vi "Communicate with Simulated Temperature Control.vi"(5 "error in (no error)":errorcluster, 6 "stop":bool, 7 "Setpoint":dbl=20.0 format="%.2f", 8 "connection ID":refnum<k5>) -> (0 "error out":errorcluster, 1 "Temperature":dbl(slide) scale=0.0..100.0, 2 "Stabilized":bool, 3 "connection ID Out":refnum<k5>)   [LabVIEW 2010]
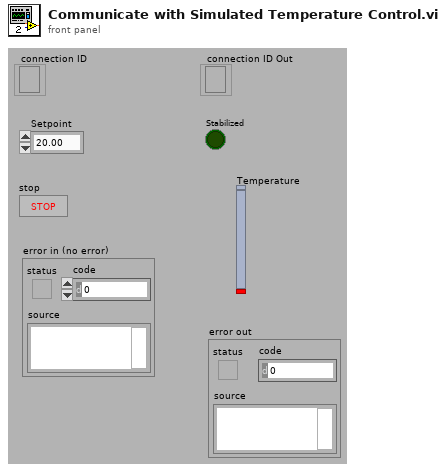
[diagram p1: front panel]
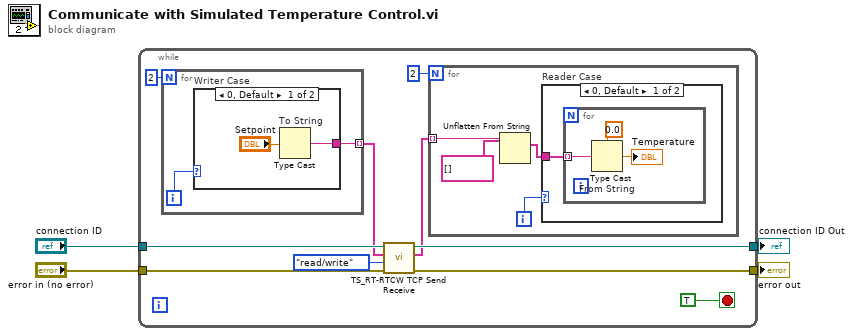
[diagram p0: block diagram]
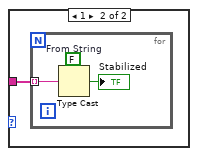
[diagram p2: hidden frame]
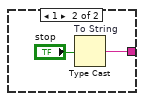
[diagram p3: hidden frame]
diagram:
  n1 = while {
    tunnel: [w13] -> w2
    tunnel: "connection ID" -> [w12]
    tunnel: "error in (no error)" -> [w14]
    tunnel: [w9] -> w4
    stop <- TRUE stop-if-true
    n2 = for {
      N: 2 -> [_]
      tunnel: [w27] -> w10 mode=indexing
      i -> [w28]
      n3 = case "Writer Case" shown="0, Default" w28 {
        tunnel: [w30 w32] -> w27
        frame 0, Default {
          n4 = Type Cast "To String"(x="Setpoint") -> (*(type *) &x=w30:string)  [unwired: 1 out]
        }
        frame 1 {
          n5 = Type Cast "To String"(x="stop") -> (*(type *) &x=w32:string)  [unwired: 1 out]
        }
      }
    }
    n6 = call "TS_RT-RTCW TCP Send Receive.vi"("error in (no error)"=w14, "access (read/write)"=enum16{"read/write", "read only", "write only"}."read/write", "Data In"=w10, "connection ID"=w12) -> ("error out"=w9:errorcluster, "Data Out"=w11:string[], "connection ID Out"=w13:refnum<k5>)  [unwired: 1 out]
    n7 = for {
      N: 2 -> [_]
      tunnel: w11 -> [w16] mode=indexing
      i -> [w18]
      n8 = Unflatten From String(type=string[] [] ("Data Out"), binary string=w16) -> (value=w15:string[])  [unwired: 1 in, 4 out]
      n9 = case "Reader Case" shown="0, Default" w18 {
        tunnel: w15 -> [w19 w23]
        frame 0, Default {
          n10 = for {
            tunnel: w19 -> [w22] mode=indexing
            n11 = Type Cast "From String"(type=0.0 ("Temperature"), x=w22) -> (*(type *) &x=→"Temperature":dbl)
          }
        }
        frame 1 {
          n12 = for {
            tunnel: w23 -> [w26] mode=indexing
            n13 = Type Cast "From String"(type=FALSE ("Stabilized"), x=w26) -> (*(type *) &x=→"Stabilized":bool)
          }
        }
      }
    }
  }
  "error out" <- w4
  "connection ID Out" <- w2
